vi "Configure Channel.vi"(8 "error in (no error)":errorcluster, 10 "DAQmx Task In":refnum<k21>, 11 "CurrentInChannel in":refnum<class "CurrentInChannel.lvclass">) -> (0 "error out":errorcluster, 2 "DAQmx Task":refnum<k21>)   [LabVIEW 2020, in "VolatusDAQConfig.lvlib" / "CurrentInChannel.lvclass"]
uses:
  CurrentInChannel.lvclass
  CurrentInChannel.lvclass/CurrentInChannel.ctl
  VolatusConfig/VolatusConfigElement/VolatusConfigElement.lvclass
  VolatusConfig/Channel/Channel Config.lvclass
  C:/dev/lv20CE/relink/lv-volatus/VolatusDAQConfig/DAQmxChannel/DAQmxChannel.lvclass
  C:/dev/lv20CE/relink/lv-volatus/VolatusConfig/Channel/Channel Config.lvclass
  C:/dev/lv20CE/relink/lv-volatus/VolatusConfig/VolatusConfigElement/VolatusConfigElement.lvclass
  C:/dev/lv20CE/relink/lv-volatus/VolatusDAQConfig/CurrentInChannel/CurrentInChannel.lvclass
  <vilib>/DAQmx/create/channels.llb/DAQmx Create Channel (AI-Current-Basic).vi
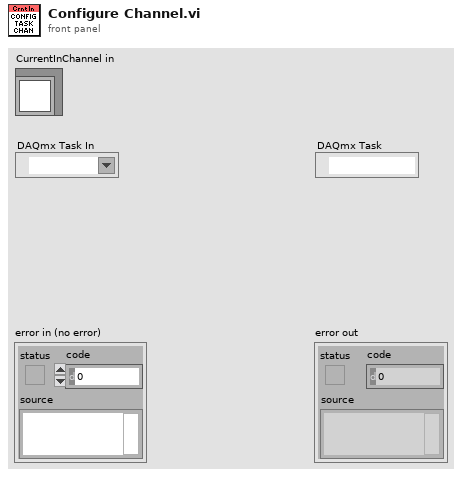
[diagram p1: front panel]
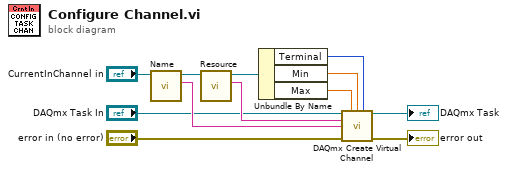
[diagram p0: block diagram]
diagram:
  n1 = call "Name.vi"("VolatusConfigElement in"="CurrentInChannel in") -> ("Name"=w6:string, "VolatusConfigElement out"=w7:refnum<class "CurrentInChannel.lvclass">)  [unwired: 8 in, 1 out]
  n2 = call "Resource.vi"("Channel in"=w7) -> ("Resource"=w8:string, "Channel out"=w9:refnum<class "CurrentInChannel.lvclass">)  [unwired: 8 in, 1 out]
  n3 = Unbundle By Name(w9) -> ("Terminal"=w12:i32, "Min"=w11:dbl, "Max"=w10:dbl)
  n4 = call-poly <vilib>:"DAQmx Create Virtual Channel.vi"("task in"="DAQmx Task In", "maximum value"=w10, "minimum value"=w11, "input terminal configuration"=w12, "physical channels"=w8, "name to assign"=w6, "error in"="error in (no error)") -> ("task out"=→"DAQmx Task":refnum<k21>, "error out"=→"error out":errorcluster)  [unwired: 7 in]
